vi "Win32 Get Error Description.vi"(8 "error in (no error)":errorcluster, 11 "current VI's path":path) -> (0 "error out":errorcluster={"status"=FALSE, "code"=0, "source"="\r\n"}, 2 "error discription":string, 3 "error code":u32)   [LabVIEW 2013]
doc: "This VI retrieves the calling VI's last error code and provides a useful description of the error that occured. This error information is bundled into <b>error out</b>, and the error status is set to True."
uses:
  kernel32.dll
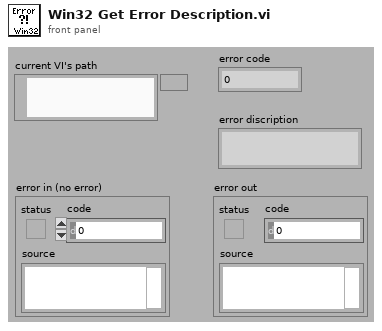
[diagram p1: front panel]
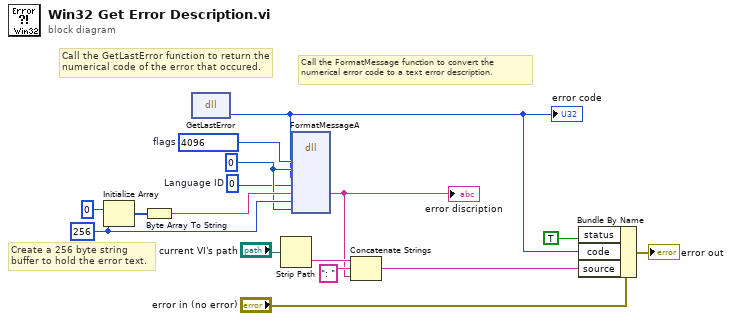
[diagram p0: block diagram]
diagram:
  w14 = u32 256 ("dimension size")
  w10 = u32 0 ("lpSource")
  w9 = u32 0  # Language ID
  w8 = u32 4096  # flags
  # "Call the FormatMessage function to convert the numerical error code to a text error description."
  # "Call the GetLastError function to return the numerical code of the error that occured."
  # "Create a 256 byte string buffer to hold the error text."
  n1 = Initialize Array(u8 0 ("element"), w14) -> (w11:u8[])
  n2 = Byte Array To String(unsigned byte array=w11) -> (string=w13:string)
  n3 = dll-call lib="kernel32.dll" fn="GetLastError"() -> ("error"=w1:u32)  [unwired: 3 in, 2 out]
  "error code" <- w1
  n4 = Strip Path(path="current VI's path") -> (name=w5:string)  [unwired: 1 out]
  n5 = dll-call lib="kernel32.dll" fn="FormatMessageA"("dwFlags"=w8, "lpSource"=w10, "dwMessageId"=w1, "dwLanguageId"=w9, "lpBuffer"=w13, "nSize"=w14, "Arguments"=w10) -> ("lpBuffer"=w3:string)  [unwired: 10 in, 2 out]
  "error discription" <- w3
  n6 = Concatenate Strings(w5, ": " ("string"), w3) -> (w2:string)
  n7 = Bundle By Name(cluster="error in (no error)", "status"=TRUE, "code"=w1, "source"=w2) -> (→"error out":errorcluster)
